vi "ap set error blink threshold.vi"(10 "delta_threshold":u32, 11 "ap_handle":u32) -> (2 "function return":i32, 3 "ap_handle out":u32)   [LabVIEW 2019, in "apdm.lvlib"]
doc: "APDM_EXPORT int apdm_ap_set_error_blink_threshold(apdm_ap_handle_t ap_handle, const uint32_t delta_threshold);"
uses:
  apdm.lvlib
  Lee Lab/CP FES Walking 2018/Code/Working/LabVIEW/apdm.dll
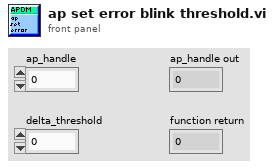
[diagram p1: front panel]
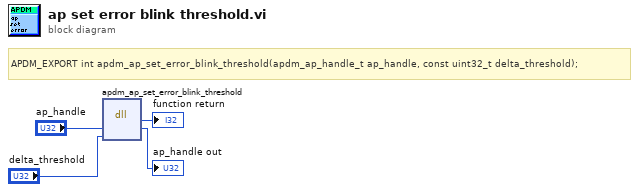
[diagram p0: block diagram]
diagram:
  # "APDM_EXPORT int apdm_ap_set_error_blink_threshold(apdm_ap_handle_t ap_handle, const uint32_t delta_threshold);"
  n1 = dll-call lib="C:/Users/jfalesi/Dropbox/Lee Lab/CP FES Walking 2018/Code/Working/LabVIEW/apdm.*" fn="apdm_ap_set_error_blink_threshold"("ap_handle"="ap_handle", "delta_threshold"="delta_threshold") -> (→"function return":i32, "ap_handle"=→"ap_handle out":u32)  [unwired: 4 in, 2 out]
